vi "Start Sync.vi"(8 "error in (no error)":errorcluster, 10 "MeasurementPlugin in":refnum<class "Measurement Plugin Service.lvclass">, 11 "IMeasurementService in":refnum<class "IMeasurement Service.lvclass">) -> (0 "error out":errorcluster, 3 "IMeasurementService out":refnum<class "IMeasurement Service.lvclass">)   [LabVIEW 2020, in "MeasurementLink Measurement Server.lvlib" / "IMeasurement Service.lvclass"]
uses:
  IMeasurement Service.lvclass
  Measurement Plugin Service/Measurement Plugin Service.lvclass
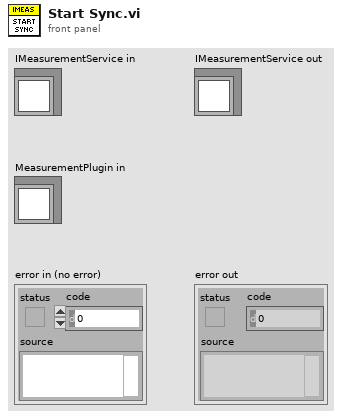
[diagram p1: front panel]
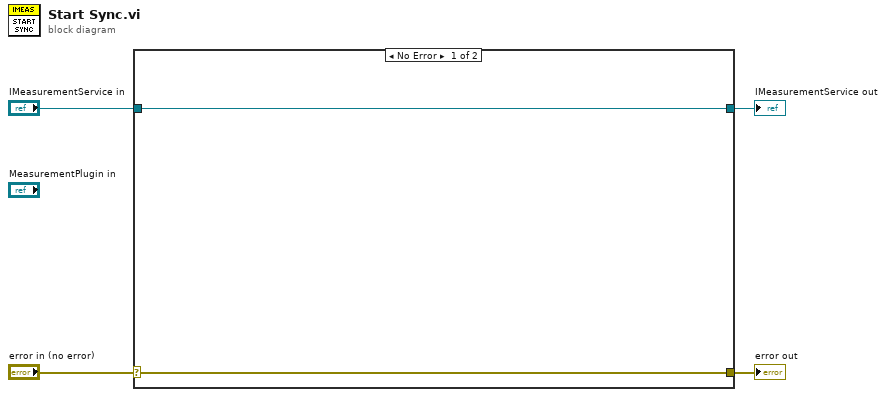
[diagram p0: block diagram]
diagram:
  n1 = case shown="No Error" "error in (no error)" {
    selector: "error in (no error)" -> [w5 w8]
    tunnel: [w5 w8] -> w3
    tunnel: [w6 w7] -> w1
    tunnel: "IMeasurementService in" -> [w6 w7]
    frame No Error {
    }
    frame Error {
    }
  }
  "error out" <- w3
  "IMeasurementService out" <- w1
